vi "Build Path__ogtk.vi"   [LabVIEW 2016]
doc: "Functions identically to LabVIEW \"Build Path\" function, but is polymorphic to also allow the path and/or input to be an array. There are two array modes:\n(1) if \"base path\" and \"name or relative path\" are arrays then the output array is built element by element with the ideces of base path corresponding to those of \"name or relative path\"\n(2) if \"base path\" is a literal and \"name or relative path\" is an array then the output array is build by appending each element in \"name or relative path\" onto base path."
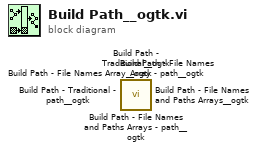
[diagram p0: block diagram]
diagram:
  n1 = call <userlib>:"Build Path - File Names and Paths Arrays - path__ogtk.vi"() -> ()  [unwired: 2 in, 1 out]
  n2 = call <userlib>:"Build Path - File Names Array - path__ogtk.vi"() -> ()  [unwired: 2 in, 1 out]
  n3 = call <userlib>:"Build Path - Traditional - path__ogtk.vi"() -> ()  [unwired: 2 in, 1 out]
  n4 = call <userlib>:"Build Path - File Names and Paths Arrays__ogtk.vi"() -> ()  [unwired: 2 in, 1 out]
  n5 = call <userlib>:"Build Path - File Names Array__ogtk.vi"() -> ()  [unwired: 2 in, 1 out]
  n6 = call <userlib>:"Build Path - Traditional__ogtk.vi"() -> ()  [unwired: 2 in, 1 out]
